vi "Schreiben_verknuepfen_Text.vi"(8 "error in (no error)":errorcluster caption="Fehler (Eingang, kein Fehler)", 9 "Order":string, 11 "parameter":string) -> (0 "error out":errorcluster caption="Fehler (Ausgang)", 3 "Verknüpfter String":string)   [LabVIEW 2020, in "Linearisierung v2.lvlib" / "Gasteiler.lvlib" / "HovaCAL_Interface.lvlib" / "KGN.lvlib"]
uses:
  KGN.lvlib
panel:
  in  "Zieladresse":string="FF"
  in  "Quelladresse":string="00"
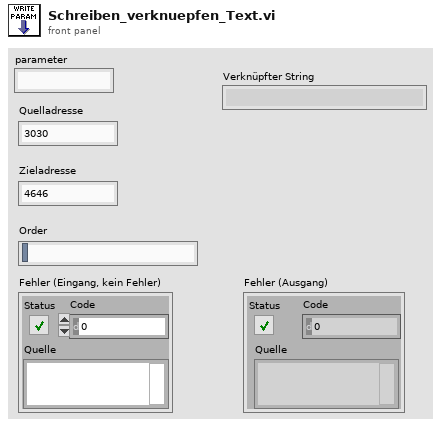
[diagram p1: front panel]
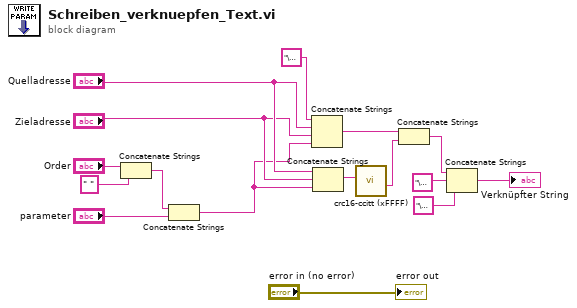
[diagram p0: block diagram]
diagram:
  n1 = Concatenate Strings("Order", " " ("String")) -> (w4:string)
  n2 = Concatenate Strings(w4, "parameter") -> (w5:string)
  n3 = Concatenate Strings("\u0002", "Quelladresse", "Zieladresse", w5) -> (w10:string)
  n4 = Concatenate Strings("Quelladresse", "Zieladresse", w5) -> (w8:string)
  n5 = call "crc16-ccitt (xFFFF).vi"("Message"=w8) -> ("Hex-Integer-String"=w7:string)  [unwired: 8 in, 2 out]
  n6 = Concatenate Strings(w10, w7) -> (w13:string)
  n7 = Concatenate Strings(w13, "\u0003", "\u0006" ("String")) -> (→"Verknüpfter String":string)
  "error out" <- "error in (no error)"
